vi "Read_Digital_Outputs_CVT.vi"() -> ()   [LabVIEW 2016, in "MB Master.lvlib"]
uses:
  <vilib>/NI/Current Value Table/DataTypes/Boolean_Read.vi
  <vilib>/NI/Current Value Table/Type to Enum.vi
  <vilib>/NI/Current Value Table/DataTypes/Boolean_Type To Enum.vi
  <vilib>/Utility/file.llb/Read Delimited Spreadsheet (string).vi
  <vilib>/NI/Current Value Table/FGVs/CVT Globals.vi
  <vilib>/NI/Current Value Table/FGVs/Tag Memory.vi
  <vilib>/NI/Current Value Table/Memory Block.vi
  <vilib>/NI/Current Value Table/DataTypes/Boolean_Memory Block.vi
  MB Master.lvlib
  <vilib>/NI/Current Value Table/Current Value Table.lvlib
panel:
  out "Array 2":cluster{"Tag Name":string, "Value":bool}[](array[cluster])
  in  "stop":bool
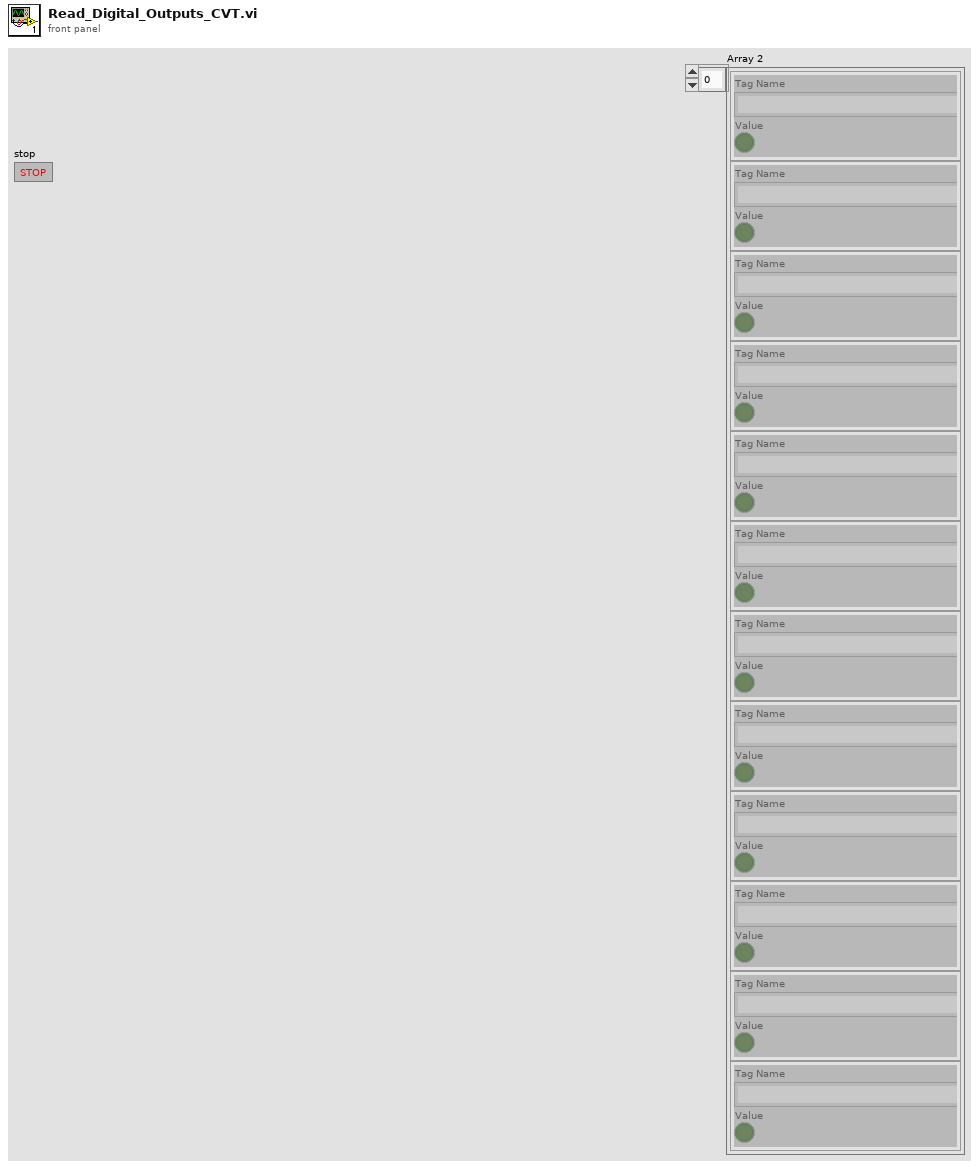
[diagram p1: front panel]
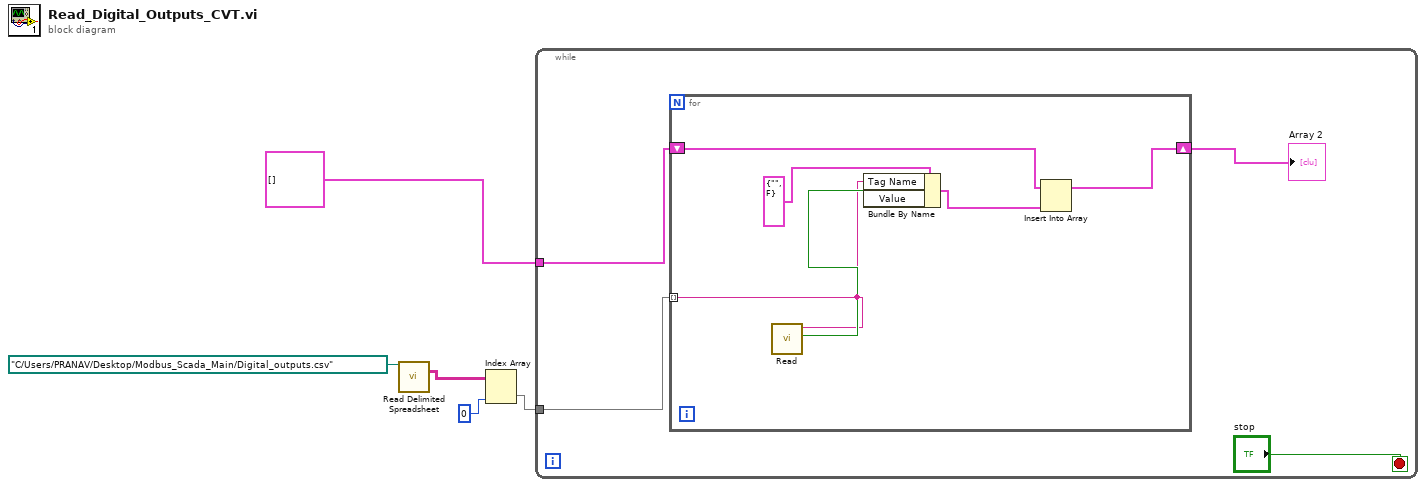
[diagram p0: block diagram]
diagram:
  n1 = call-poly <vilib>:"Read Delimited Spreadsheet.vi"("file path (dialog if empty)"=path "C:/Users/PRANAV/Desktop/Modbus_Scada_Main/Digital_outputs.csv") -> ("all rows"=w1:string[][])  [unwired: 9 in, 5 out]
  n2 = Index Array "Index Array"(array=w1, index (col)=0 ("disabled index (col)")) -> (element=w3:string[])  [unwired: 1 in]
  n3 = while {
    tunnel: cluster{"Tag Name":string, "Value":bool}[] [] ("output array") -> [w8]
    tunnel: w3 -> [w6]
    stop <- "stop" stop-if-true
    n4 = for {
      shift-right: [w15] -> w9
      shift-left: w8 -> [w10]
      tunnel: w6 -> [w11] mode=indexing
      n5 = call-poly <vilib>:"Read.vi"("Tag Name"=w11) -> ("Value"=w12:bool)  [unwired: 9 in, 1 out]
      n6 = Bundle By Name(cluster=cluster{"Tag Name":string, "Value":bool} {"Tag Name"="", "Value"=FALSE} ("Cluster"), "Tag Name"=w11, "Value"=w12) -> (w13:cluster{"Tag Name":string, "Value":bool})
      n7 = Insert Into Array "Insert Into Array"(array=w10, new element=w13) -> (w15:cluster{"Tag Name":string, "Value":bool}[])  [unwired: 1 in]
    }
    "Array 2" <- w9
  }
